vi "flow-builder-nutrition-check.vi"(7 "clk":dbl) -> (0 "error out":errorcluster, 2 "Check Report":string, 3 "intructions out":variant[](array[variant]))   [LabVIEW 2024]
uses:
  controls/UiStepBuilder.ctl
  controls/type.step-builder.ctl
  build.flowToVarient.vi
  <vilib>/Utility/error.llb/Trim Whitespace.vi
  Polymorphics/variantCtrl.polymorphic.vi
  Polymorphics/variantCtrlStepFunction.vi
  Polymorphics/variantCtrlSetpoint.vi
  Polymorphics/variantCtrlString.vi
  proc.util.enumToStrStepVar.vi
  Polymorphics/variantCtrlNumber.vi
  util.DelimitedStringToArray.vi
  <vilib>/Utility/error.llb/Trim Whitespace One-Sided.vi
  proc.util.validateParamExist.vi
  <vilib>/Utility/error.llb/Clear Errors.vi
  globals/globals-engine.vi
  build.elementToParamString.vi
  util.error.create.vi
  Polymorphics/variantCtrlStepPointer.vi
  Polymorphics/variantCtrlStepUserMessage.vi
  Polymorphics/variantCtrlStepPath.vi
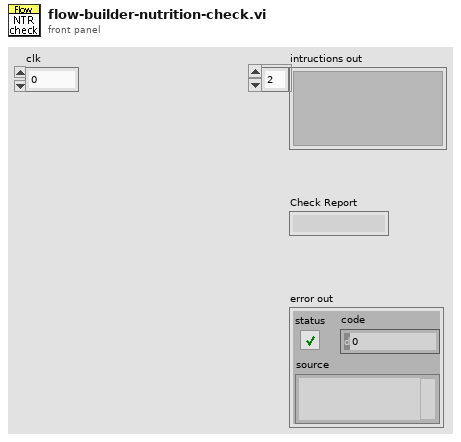
[diagram p1: front panel]
types:
  T1 = typedef "UiNutritionPanel.ctl" = cluster{"Main":cluster{"Enable":bool, "WashTimes":cluster{"In":dbl, "Out":dbl}, "DailyActivityHours":cluster{"Begin Time":T2, "End Time":T2}[]}, "Water Dosing":cluster{"Water Dose":dbl, "Water Limit":dbl}, "EC Ranges":cluster{"H Alarm":dbl, "L Alarm":dbl, "Low":dbl}, "EC Dosing":cluster{"ALFA1 Dose":dbl, "ALFA1 Limit":dbl, "BETA1 Dose":dbl, "BETA1 Limit":dbl, "ALFA2 Dose":dbl, "ALFA2 Limit":dbl, "BETA2 Dose":dbl, "BETA2 Limit":dbl}, "PH Ranges":cluster{"H Alarm":dbl, "L Alarm":dbl, "High":dbl, "Low":dbl}, "PH Dosing":cluster{"ACID Dose":dbl, "ACID Limit":dbl, "BASE Dose":dbl, "BASE Limit":dbl}, "ORP Ranges":cluster{"H Alarm":dbl, "L Alarm":dbl, "Low":dbl}, "ORP Dosing":cluster{"MIX Dose":dbl, "MIX Limit":dbl}}
  T2 = typedef "UiScheduleTimestamp.ctl" = timestamp
  T3 = typedef "type.step-builder.ctl" = enum16{"NO_OPERATION", "DELAY-JUMP", "DELAY", "JUMP", "COMPLETE", "SCHEDULER", "IRR-CHECK", "UNIT-CHECK", "UNIT-SAMPLE", "UNIT-DOSE", "LOG-REPORT", "LOG-MESSAGE", "IO-READ", "IO-READ-MANY", "IO-WRITE", "IO-COMPARE-OUT", "IO-COMPARE-IN", "PROC-START", "PROC-STOP", "PROC-LOAD", "PROC-IS-COMPLETED", "RECORD-MOVE", "GET-RH", "GET-UV", "GET-WD", "GET-WS", "OCS-CHECK", "OCS-RECORD"}
  T4 = typedef "UiStepBuilder.ctl" = cluster{"Step Function":T3, "ParamString":string, "Step Label":string}
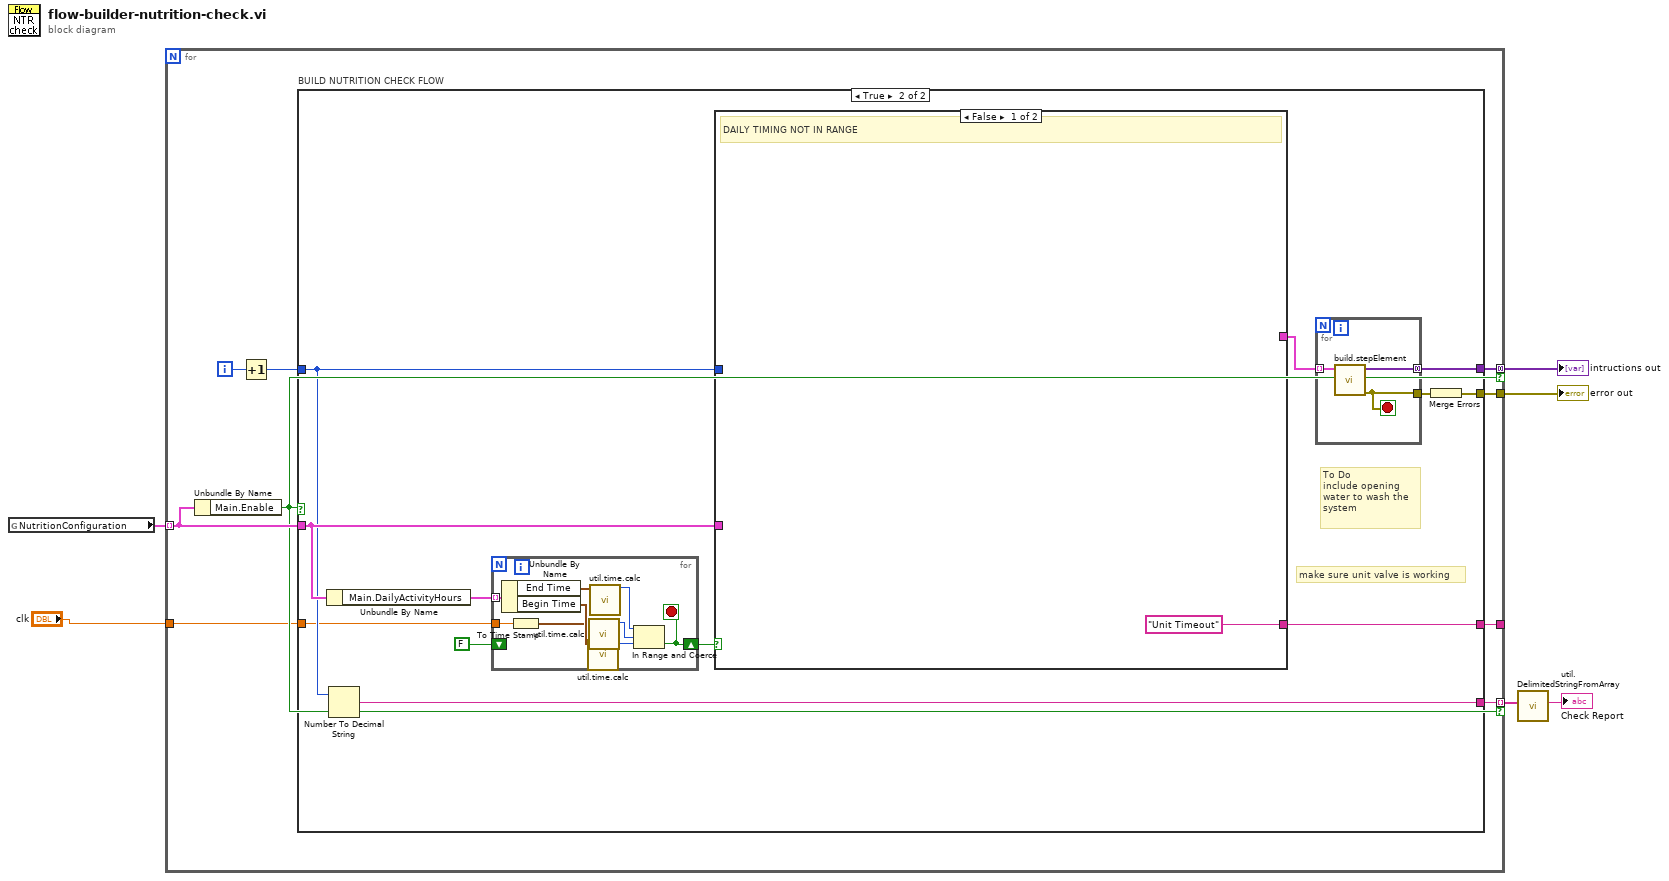
[diagram p0: block diagram]
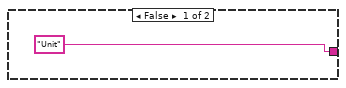
[diagram p2: hidden frame]
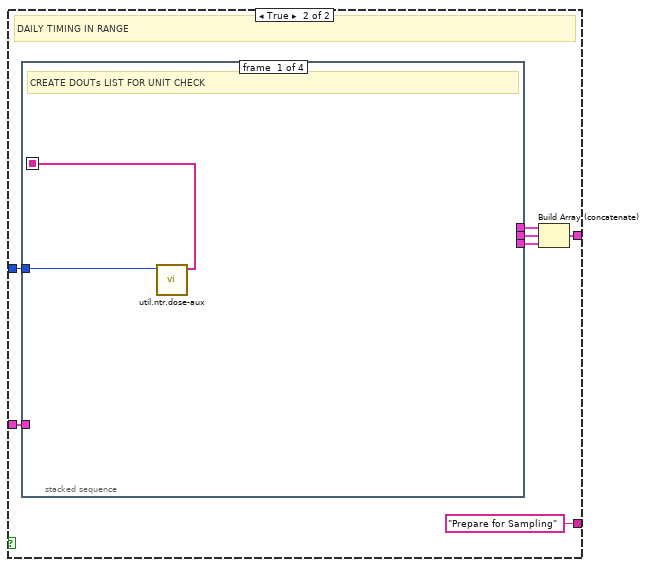
[diagram p3: hidden frame]
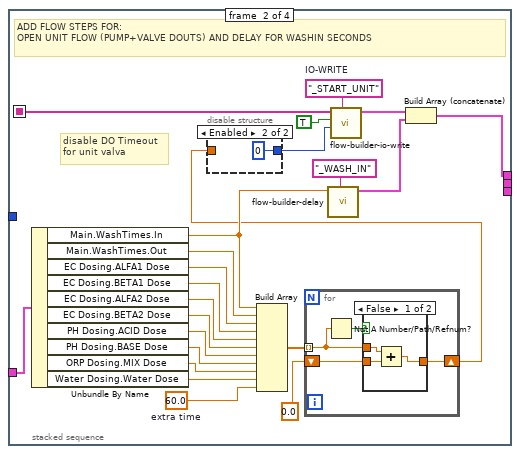
[diagram p4: hidden frame]
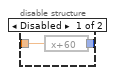
[diagram p5: hidden frame]
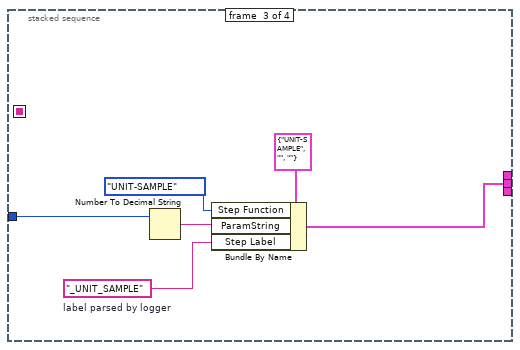
[diagram p7: hidden frame]
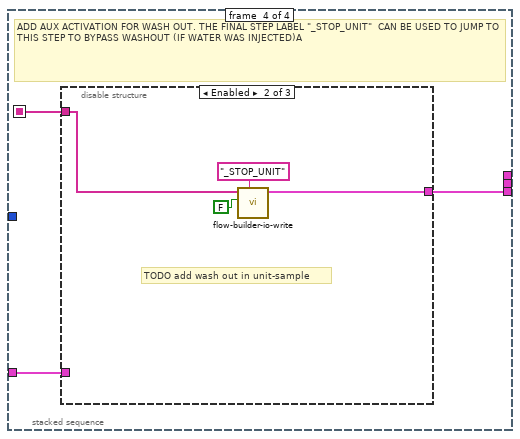
[diagram p8: hidden frame]
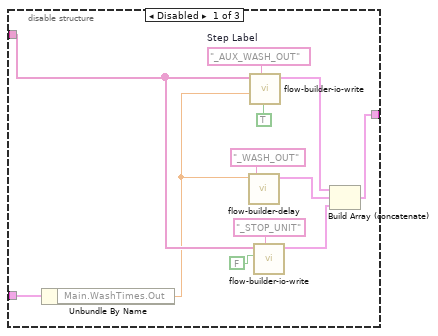
[diagram p9: hidden frame]
diagram:
  n1 = global read "globals-engine.vi" "NutritionConfiguration"() -> (w4:T1[])
  n2 = for {
    tunnel: [w15] -> w6 mode=concatenating if=w8
    tunnel: [w14] -> w5
    tunnel: [w13] -> _
    tunnel: w4 -> [w12] mode=indexing
    tunnel: [w9] -> w3 mode=indexing if=w8
    tunnel: "clk" -> [w7]
    i -> [w11]
    n3 = Unbundle By Name(w12) -> ("Main.Enable"=w8:bool)
    n4 = Increment(x=w11) -> (x+1=w10:i32)
    n5 = case "BUILD NUTRITION CHECK FLOW" shown="True" w8 {
      tunnel: [_ w28] -> w15
      tunnel: [_ w27] -> w14
      tunnel: w10 -> [_ w19]
      tunnel: w12 -> [_ w25]
      tunnel: ["Unit" w21] -> w13
      tunnel: [_ w18] -> w9
      tunnel: w7 -> [_ w17]
      frame False {
      }
      frame True {
        # "make sure unit valve is working"
        # "To Do \ninclude opening\nwater to wash the \nsystem"
        n6 = Unbundle By Name(w25) -> ("Main.DailyActivityHours"=w24:cluster{"Begin Time":T2, "End Time":T2}[])
        n7 = Number To Decimal String(number=w19) -> (decimal integer string=w18:string)  [unwired: 1 in]
        n8 = for {
          tunnel: w24 -> [w106] mode=indexing
          tunnel: w17 -> [w102]
          shift-right: [w98] -> w22
          shift-left: FALSE -> [_]
          stop <- w98 stop-if-true
          n9 = Unbundle By Name(w106) -> ("End Time"=w105:T2, "Begin Time"=w103:T2)
          n10 = To Time Stamp(1:w102) -> (0:w101:timestamp)
          n11 = call "util.time.calc.vi"("Begin Time"=w103) -> ("daily seconds counter"=w104:i32)  [unwired: 10 in]
          n12 = call "util.time.calc.vi"("Begin Time"=w101) -> ("daily seconds counter"=w100:i32)  [unwired: 10 in]
          n13 = call "util.time.calc.vi"("Begin Time"=w105) -> ("daily seconds counter"=w99:i32)  [unwired: 10 in]
          n14 = In Range and Coerce(upper limit=w99, x=w100, lower limit=w104) -> (In Range?=w98:bool)  [unwired: 1 out]
        }
        n15 = case shown="False" w22 {
          tunnel: w19 -> [_ w36]
          tunnel: w25 -> [_ w35]
          tunnel: [_ w31] -> w20
          tunnel: ["Unit Timeout" "Prepare for Sampling"] -> w21
          frame False {
            # "DAILY TIMING NOT IN RANGE"
          }
          frame True {
            # "DAILY TIMING IN RANGE"
            n16 = stacked-sequence {
              seq-local: [w37 _ _ _] -> [_ w54 _ w81]
              tunnel: w36 -> [w38 _ w75 _]
              tunnel: w35 -> [_ w61 _ w80]
              tunnel: [_ w53 _ _] -> w34
              tunnel: [_ _ w74 _] -> w33
              tunnel: [_ _ _ w79] -> w32
              frame #0 {
                # "CREATE DOUTs LIST FOR UNIT CHECK"
                n17 = call "util.ntr.dose-aux.vi"("Unit Index"=w38) -> ("DO Unit Pumps"=w37:string[])  [unwired: 6 in, 4 out]
              }
              frame #1 {
                w42 = 60.0  # extra time
                w55 = "_START_UNIT"  # IO-WRITE
                # "disable DO Timeout\nfor unit valva"
                # "ADD FLOW STEPS FOR:\nOPEN UNIT FLOW (PUMP+VALVE DOUTS) AND DELAY FOR WASHIN SECONDS"
                n18 = Unbundle By Name(w61) -> ("Main.WashTimes.In"=w43:dbl, "Main.WashTimes.Out"=w44:dbl, "EC Dosing.ALFA1 Dose"=w45:dbl, "EC Dosing.BETA1 Dose"=w46:dbl, "EC Dosing.ALFA2 Dose"=w47:dbl, "EC Dosing.BETA2 Dose"=w48:dbl, "PH Dosing.ACID Dose"=w49:dbl, "PH Dosing.BASE Dose"=w50:dbl, "ORP Dosing.MIX Dose"=w51:dbl, "Water Dosing.Water Dose"=w52:dbl)
                n19 = Build Array(w43, w44, w45, w46, w47, w48, w49, w50, w51, w52, w42) -> (w41:dbl[])
                n20 = for {
                  tunnel: w41 -> [w65] mode=indexing
                  shift-right: [w68] -> w39
                  shift-left: 0.0 ("element") -> [w67]
                  n21 = Not A Number/Path/Refnum?(number/path/refnum=w65) -> (NaN/Path/Refnum?=w66:bool)
                  n22 = case shown="False" w66 {
                    tunnel: w65 -> [w71 _]
                    tunnel: [w70 w72] -> w68
                    tunnel: w67 -> [w69 w72]
                    frame False {
                      n23 = Add(x=w71, y=w69) -> (x+y=w70:dbl)
                    }
                    frame True {
                    }
                  }
                }
                n24 = disable-structure shown="Enabled" {
                  disable-tunnel: [w63 u16 0 ("Digital Timeout")] -> w60
                  disable-tunnel: w39 -> [w62 _]
                  frame Disabled {
                    n25 = expression code="x+60"(w62) -> (w63:dbl)
                  }
                  frame Enabled {
                  }
                }
                n26 = call "flow-builder-delay.vi"("Step Label"="_WASH_IN", "Delay [s]"=w43) -> ("Step Element"=w59:T4)  [unwired: 9 in]
                n27 = call "flow-builder-io-write.vi"("Step Name"=w55, "Digital Timeout"=w60, "Value in"=TRUE ("UiDeviceConstant"), "Dout+AUX"=w54) -> ("Flow out"=w57:T4[])  [unwired: 7 in]
                n28 = Build Array (concatenate)(w57, w59) -> (w53:T4[])
              }
              frame #2 {
                w73 = "_UNIT_SAMPLE"  # label parsed by logger
                n29 = Number To Decimal String(number=w75) -> (decimal integer string=w77:string)  [unwired: 1 in]
                n30 = Bundle By Name(cluster=T4 {"Step Function"=enum."UNIT-SAMPLE", "ParamString"="", "Step Label"=""} ("FlowModeConstant 2"), "Step Function"=type.step-builder."UNIT-SAMPLE" ("UiStepFunction"), "ParamString"=w77, "Step Label"=w73) -> (w74:T4)
              }
              frame #3 {
                # "ADD AUX ACTIVATION FOR WASH OUT. THE FINAL STEP LABEL \"_STOP_UNIT\"  CAN BE USED TO JUMP TO THIS STEP TO BYPASS WASHOUT (IF WATER WAS INJECTED)A"
                n31 = disable-structure shown="Enabled" {
                  disable-tunnel: w81 -> [w87 w95 _]
                  disable-tunnel: w80 -> [w86 _ _]
                  disable-tunnel: [w85 w94 _] -> w79
                  frame Disabled {
                    w89 = "_AUX_WASH_OUT"  # Step Label
                    n32 = Unbundle By Name(w86) -> ("Main.WashTimes.Out"=w84:dbl)
                    n33 = call "flow-builder-delay.vi"("Step Label"="_WASH_OUT", "Delay [s]"=w84) -> ("Step Element"=w91:T4)  [unwired: 9 in]
                    n34 = call "flow-builder-io-write.vi"("Step Name"=w89, "Digital Timeout"=w84, "Value in"=TRUE ("UiDeviceConstant"), "Dout+AUX"=w87) -> ("Flow out"=w93:T4[])  [unwired: 7 in]
                    n35 = call "flow-builder-io-write.vi"("Step Name"="_STOP_UNIT" ("Step Label"), "Value in"=FALSE ("UiDeviceConstant"), "Dout+AUX"=w87) -> ("Flow out"=w92:T4[])  [unwired: 8 in]
                    n36 = Build Array (concatenate)(w93, w91, w92) -> (w85:T4[])
                  }
                  frame Enabled {
                    # "TODO add wash out in unit-sample"
                    n37 = call "flow-builder-io-write.vi"("Step Name"="_STOP_UNIT" ("Step Label"), "Value in"=FALSE ("UiDeviceConstant"), "Dout+AUX"=w95) -> ("Flow out"=w94:T4[])  [unwired: 8 in]
                  }
                  frame Disabled {
                  }
                }
              }
            }
            n38 = Build Array (concatenate)(w34, w33, w32) -> (w31:T4[])
          }
        }
        n39 = for {
          tunnel: w20 -> [w109] mode=indexing
          tunnel: [w108] -> w28 mode=concatenating
          tunnel: [w107] -> w26
          stop <- w107 stop-if-true
          n40 = call "build.stepElement.vi"("Step in"=w109) -> ("error out"=w107:errorcluster, "steps out"=w108:variant[])  [unwired: 9 in]
        }
        n41 = Merge Errors(w26) -> (w27:errorcluster)
      }
    }
  }
  "intructions out" <- w6
  "error out" <- w5
  n42 = call "util.DelimitedStringFromArray.vi"("params array in"=w3) -> ("delimited string out"=→"Check Report":string)  [unwired: 10 in]
